vi "(BAVSR) Process & Clean Channels.vi"(10 "C Array":i32[](array[numeric]), 11 "Channel Control & Legend":string[][](array[string])) -> (0 "Relevant Channel Names":string[](array[string]), 1 "Relevant Channel List":i32[](array[numeric]), 2 "Channel # Column":i32[](array[numeric]), 3 "Cleaned Channel List":string[](array[string]), 4 "Relevant Channel Label Toggles":string[](array[string]))   [LabVIEW 2023]
uses:
  1e949da2-8a3c-8c4b-8f9e-521617de89b0.vi
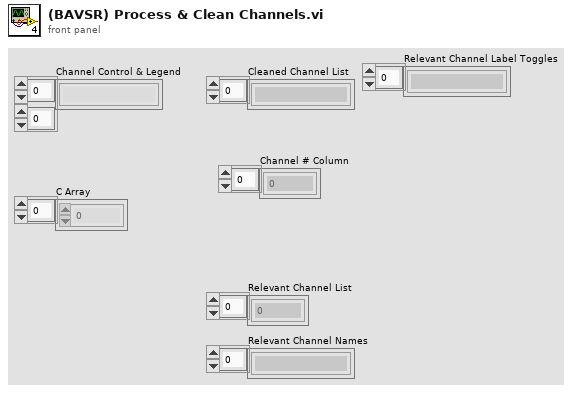
[diagram p1: front panel]
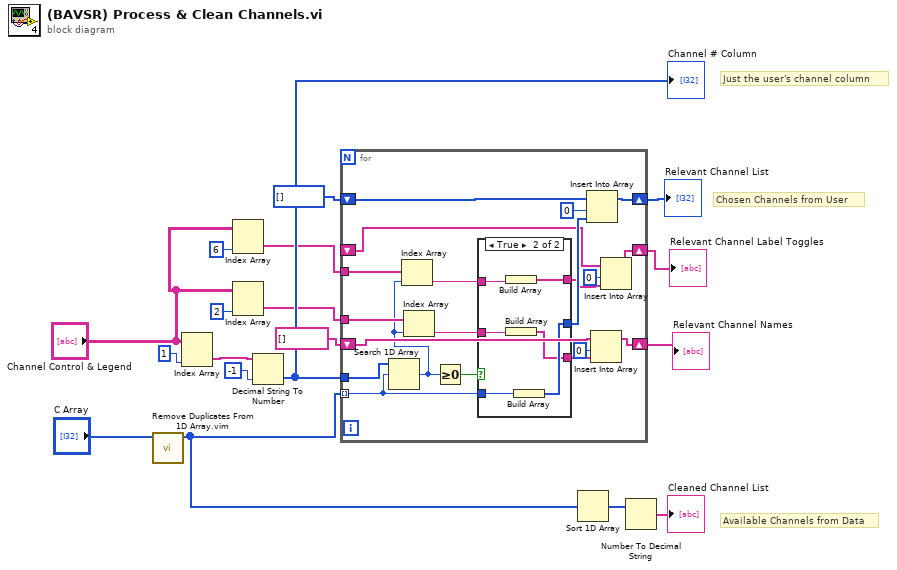
[diagram p0: block diagram]
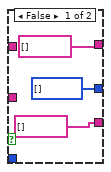
[diagram p2: hidden frame]
diagram:
  # "Just the user's channel column"
  # "Chosen Channels from User"
  # "Available Channels from Data"
  n1 = call "Remove Duplicates From 1D Array.vim"("array"="C Array") -> ("array with duplicates removed"=w15:i32[])  [unwired: 10 in]
  n2 = Index Array(array="Channel Control & Legend", index (col)=1 ("disabled index (col)")) -> (element=w14:string[])  [unwired: 1 in]
  n3 = Index Array(array="Channel Control & Legend", index (col)=6 ("disabled index (col)")) -> (element=w2:string[])  [unwired: 1 in]
  n4 = Index Array(array="Channel Control & Legend", index (col)=2 ("disabled index (col)")) -> (element=w6:string[])  [unwired: 1 in]
  n5 = Decimal String To Number(string=w14, default (0L)=-1 ("default (0 I32)")) -> (number=w9:i32[])  [unwired: 1 in, 1 out]
  "Channel # Column" <- w9
  n6 = for {
    tunnel: w9 -> [w38]
    tunnel: w15 -> [w36] mode=indexing
    shift-right: [w34] -> w16
    shift-left: i32[] [] -> [w35]
    shift-right: [w28] -> w5
    shift-left: string[] [] -> [w29]
    tunnel: w6 -> [w27]
    tunnel: w2 -> [w24]
    shift-right: [w20] -> w1
    shift-left: _ -> [w21]
    n7 = Search 1D Array(1D array=w38, element=w36) -> (index of element=w25:i32)  [unwired: 1 in]
    n8 = Index Array(array=w24, index=w25) -> (element=w23:string)
    n9 = Index Array(array=w27, index=w25) -> (element=w26:string)
    n10 = Greater Or Equal To 0?(x=w25) -> (x >= 0?=w37:bool)
    n11 = case shown="True" w37 {
      tunnel: w36 -> [_ w47]
      tunnel: [i32[] [] w46] -> w33
      tunnel: w26 -> [_ w45]
      tunnel: [string[] [] w44] -> w31
      tunnel: w23 -> [_ w43]
      tunnel: [string[] [] w42] -> w22
      frame False {
      }
      frame True {
        n12 = Build Array(w43) -> (w42:string[])
        n13 = Build Array(w45) -> (w44:string[])
        n14 = Build Array(w47) -> (w46:i32[])
      }
    }
    n15 = Insert Into Array(array=w35, index=0, new element=w33) -> (w34:i32[])
    n16 = Insert Into Array(array=w29, index=0, new element=w31) -> (w28:string[])
    n17 = Insert Into Array(array=w21, index=0, new element=w22) -> (w20:string[])
  }
  "Relevant Channel List" <- w16
  "Relevant Channel Names" <- w5
  "Relevant Channel Label Toggles" <- w1
  n18 = Sort 1D Array(array=w15) -> (sorted array=w10:i32[])
  n19 = Number To Decimal String(number=w10) -> (decimal integer string=→"Cleaned Channel List":string[])  [unwired: 1 in]
